vi "Sub Panel Status Flag_DStr-Scope SP.vi"() -> ()   [LabVIEW 2012]
panel:
  out "Config?":bool
  out "Measure?":bool
  out "Cursor?":bool
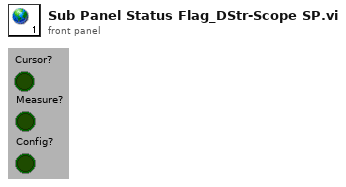
[diagram p1: front panel]
diagram:
